vi "Vision 2.vi"(0 "RGB":T1, 3 "Binary":T1, 4 "Convex":bool) -> (5 "RGB":T1, 7 "Binary":T1)   [LabVIEW 2014]
uses:
  <vilib>/vision/Image Controls.llb/IMAQ Image.ctl
  <vilib>/vision/NI_Vision_Development_Module.lvlib
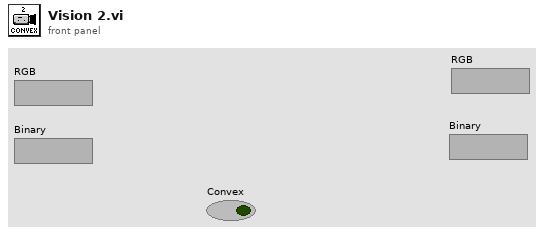
[diagram p1: front panel]
types:
  T1 = typedef "IMAQ Image.ctl" = refnum<image>
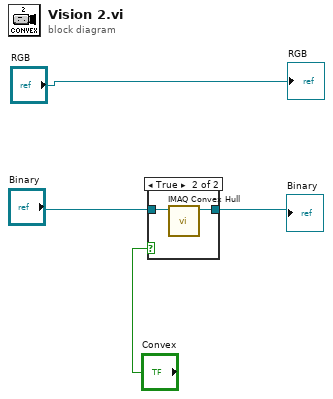
[diagram p0: block diagram]
diagram:
  n1 = case shown="True" "Convex" {
    tunnel: "Binary" -> [w5 w7]
    tunnel: [w5 w6] -> w3
    frame False {
    }
    frame True {
      n2 = call "IMAQ Convex Hull"("Image Src"=w7) -> ("Image Dst Out"=w6:T1)  [unwired: 9 in, 1 out]
    }
  }
  "Binary" <- w3
  "RGB" <- "RGB"
